vi "FileSync.Sync Config Dialog.vi"(11 "Sync Config":T1[](array[typedef])) -> (2 "OK":bool, 3 "Sync Config Out":T1[](array[typedef]))   [LabVIEW 2024, in "KATE_Lib.lvlib" / "File Utils.lvlib" / "File.Sync.lvclass"]
uses:
  File.Sync.lvclass
  File.Sync Item Record.ctl
panel:
  out "Tab Control":enum32{"Data", "Output"}(tab)
  in  "Cancel Button":bool
  in  "OK Button":bool
  # "File Sync Setup"
  # "Name/Interval/Type                                                                                                              Source/Destination"
  # "NOTES:\n - If Source is a folder then Dest must be a folder.\n - Files and subfolders are moved from the source path to the destination path.  \n    In order to move a folder from a source location to a destination location, the source and destination path must both include the folder."
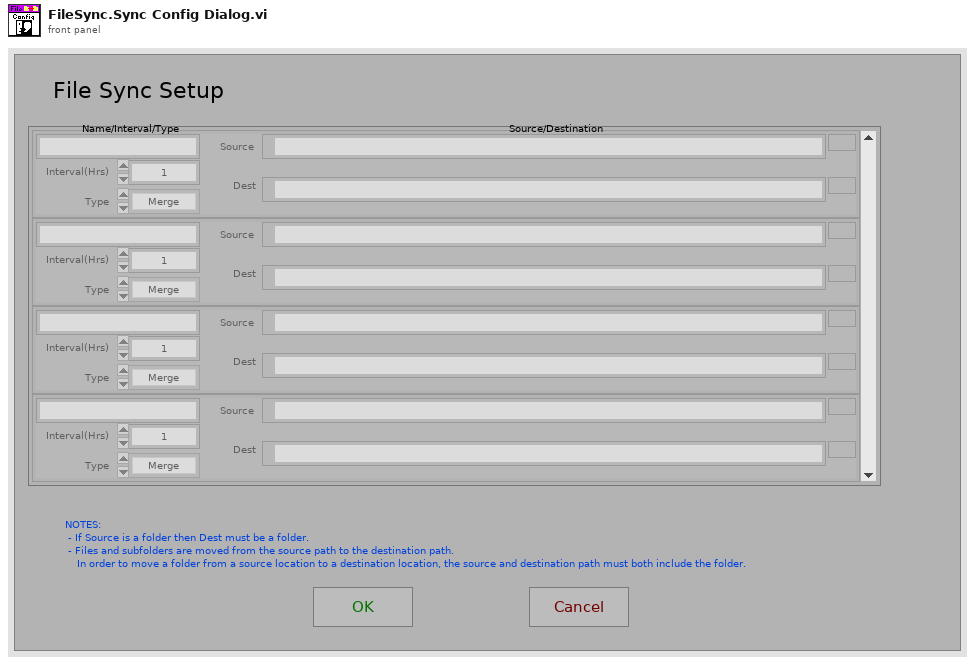
[diagram p1: front panel]
types:
  T1 = typedef "KATE_Lib.lvlib/File Utils.lvlib/File.Sync.lvclass/File.Sync Item Record.ctl" = cluster{"Name":string, "Interval":dbl, "Source":path, "Dest":path, "LastSync":timestamp, "Status":string, "Error":bool, "Type":enum16{"Merge", "Match"}}
  T2 = enum32{"Invalid", "Standard", "Closed", "Hidden", "Minimized", "Maximized"}
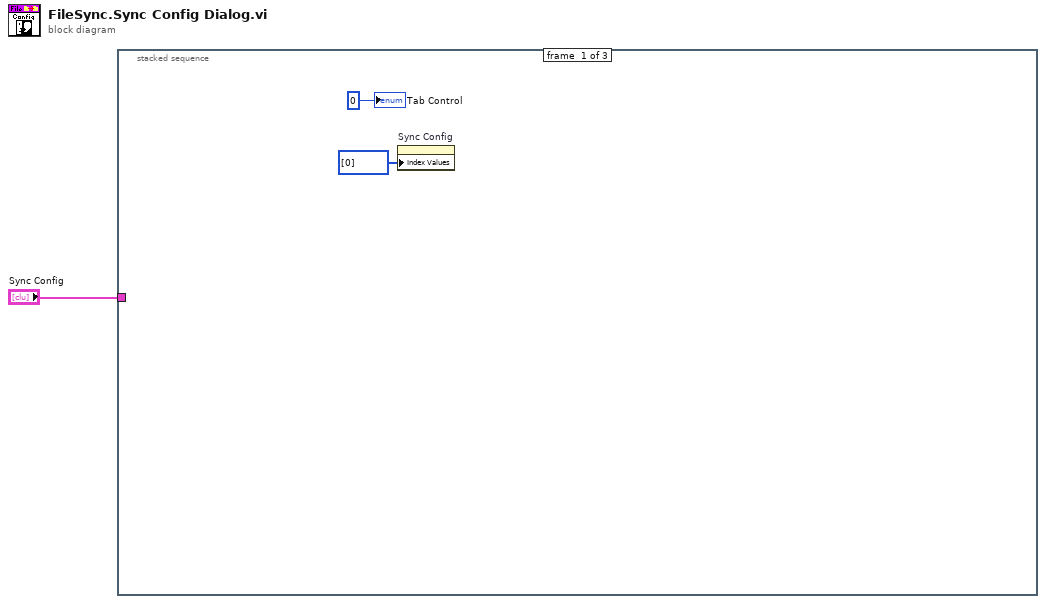
[diagram p0: block diagram]
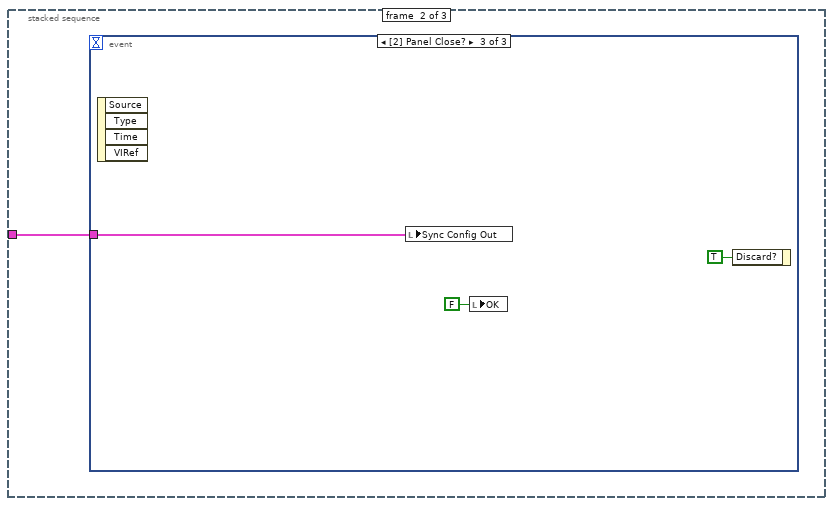
[diagram p2: hidden frame]
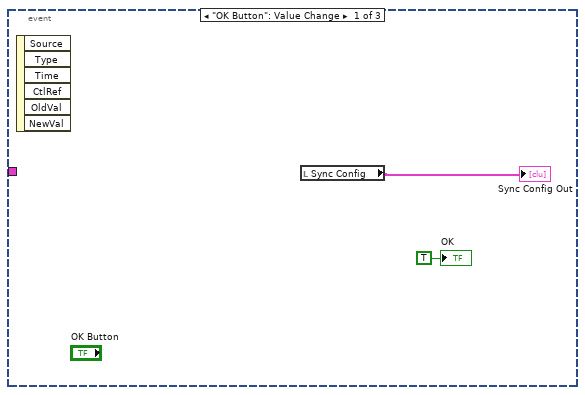
[diagram p3: hidden frame]
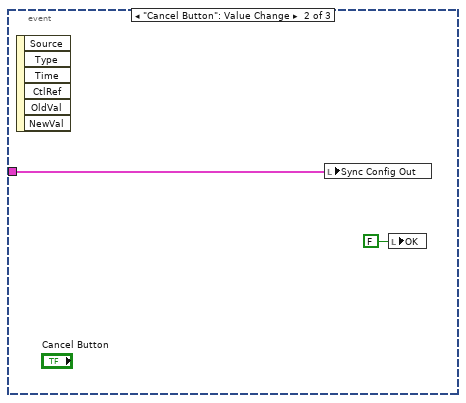
[diagram p4: hidden frame]
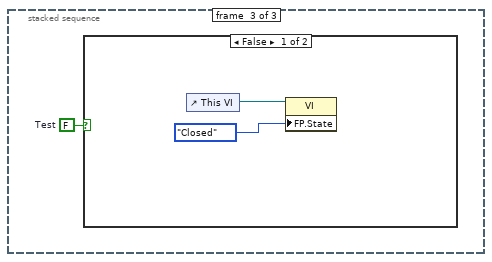
[diagram p5: hidden frame]
diagram:
  n1 = stacked-sequence {
    tunnel: "Sync Config" -> [_ w4 _]
    frame #0 {
      n2 = property on="Sync Config" class="Arr (strict)"("Index Values"=u32[] [0]) -> ()  [unwired: 2 in, 2 out]
      "Tab Control" <- 0
    }
    frame #1 {
      n3 = event shown="[2] Panel Close?" {
        selector: _ -> [_ _ _]
        dyn-events: _ -> [_ _ _]
        timeout: _ -> [_ _ _]
        tunnel: w4 -> [_ w7 w10]
        event "OK Button": Value Change {
          n4 = event-data() -> ()  [unwired: 1 in, 6 out]
          n5 = local read "Sync Config"() -> (→"Sync Config Out":T1[])
          "OK" <- TRUE ("OK")
        }
        event "Cancel Button": Value Change {
          n6 = event-data() -> ()  [unwired: 1 in, 6 out]
          n7 = local write "Sync Config Out"(w7) -> ()
          n8 = local write "OK"(FALSE ("OK")) -> ()
        }
        event Panel Close? {
          n9 = event-data() -> ()  [unwired: 1 in, 4 out]
          n10 = local write "Sync Config Out"(w10) -> ()
          n11 = local write "OK"(FALSE ("OK")) -> ()
          n12 = event-data("Discard?"=TRUE) -> ()  [unwired: 1 in, 1 out]
        }
      }
    }
    frame #2 {
      w12 = FALSE  # Test
      n13 = case shown="False" w12 {
        frame False {
          n14 = control-ref of="This VI"() -> (w14:refnum<vi>)
          n15 = property class="VI"(reference=w14, "FP.State"=T2."Closed" ("Front Panel Window:State")) -> ()  [unwired: 1 in, 2 out]
        }
        frame True {
        }
      }
    }
  }
